vi "csmdoc_load vi description map.vi"(8 "Error In":errorcluster caption="error in (no error)", 10 "Pattern":string="VI Description(CN) - *", 11 "Path":path=path "D:/CSM Framework/Communicable-State-Machine/src/help/NEVSTOP/Communicable State Machine(CSM)") -> (0 "error out":errorcluster, 2 "NoteMap":variant, 3 "DescMap":variant)   [LabVIEW 2017, in "csmdoc.lvlib"]
doc: "### csmdoc_load vi description map.vi\n\n-- <b>Controls</b> --\n- <b>Path</b>:\n\n-- <b>Indicators</b> --\n- <b>text</b>:\n- <b>variant 2</b>:\n- <b>variant</b>:"
uses:
  csmdoc.lvlib
  Communicable State Machine.lvlib
  _Shared/CSM Shared.lvlib
panel:
  out "orders":string[](array[string])
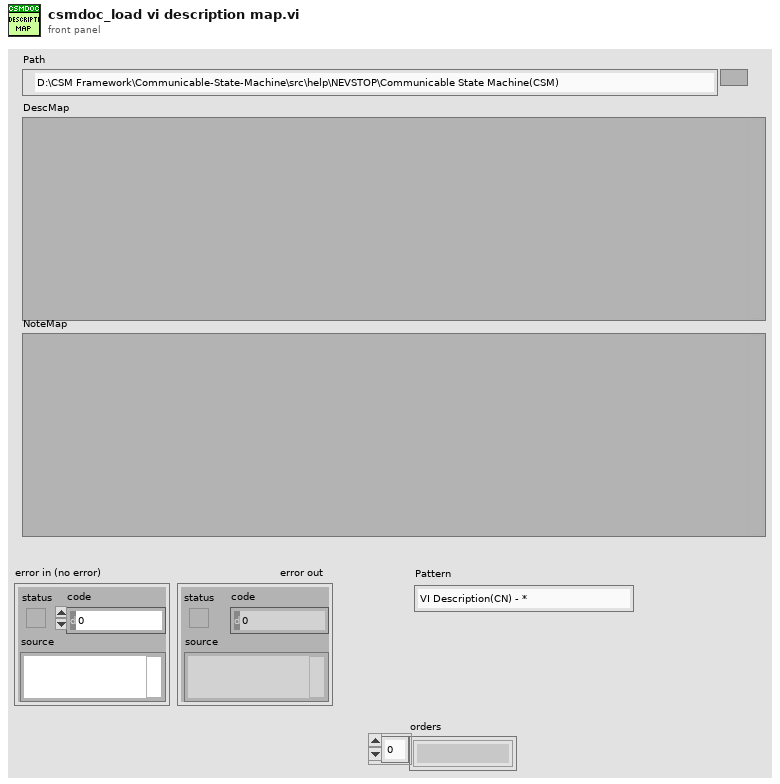
[diagram p1: front panel]
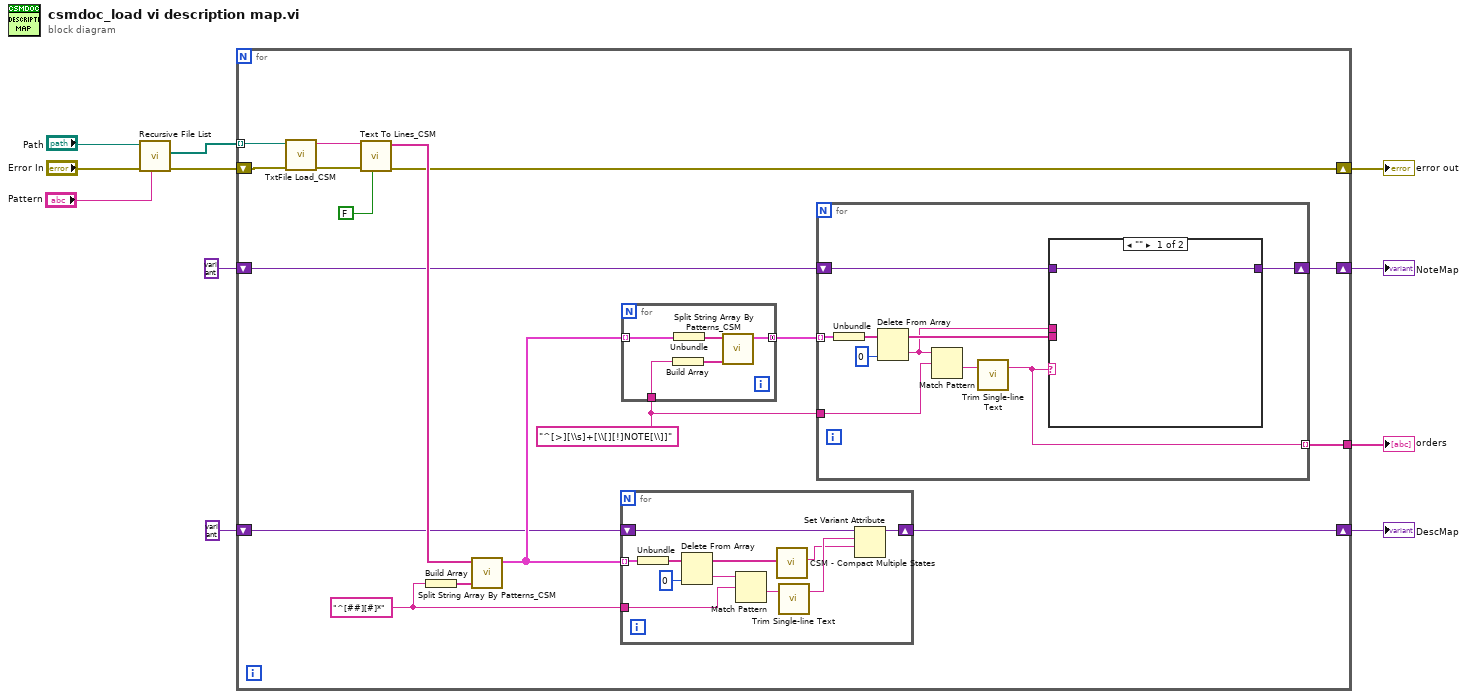
[diagram p0: block diagram]
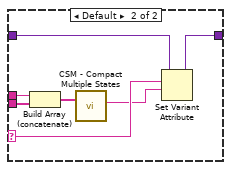
[diagram p2: hidden frame]
diagram:
  n1 = call <vilib>:"Recursive File List.vi"("pattern"="Pattern", "error in (no error)"="Error In", "Folder Path"="Path") -> ("error out"=w5:errorcluster, "All Files in Dir"=w3:path[])  [unwired: 4 in, 3 out]
  n2 = for {
    tunnel: w3 -> [w28] mode=indexing
    tunnel: [w13] -> w6
    shift-right: [w19] -> w9
    shift-left: w5 -> [w20]
    shift-right: [w14] -> w7
    shift-left: variant ("variant") -> [w17]
    shift-right: [w22] -> w11
    shift-left: variant ("variant") -> [w12]
    w15 = "^[>][\\s]+[\\[][!]NOTE[\\]]" ("delimited string")
    w24 = "^[##][#]*" ("delimited string")
    n3 = call "TxtFile Load_CSM.vi"("error in (no error)"=w20, "Path"=w28) -> ("error out"=w27:errorcluster, "Text"=w26:string)  [unwired: 8 in]
    n4 = call "Text To Lines_CSM.vi"("Remove Empty Lines? (T)"=FALSE ("Remove Empty Lines?(T)"), "error in (no error)"=w27, "String"=w26) -> ("error out"=w19:errorcluster, "Lines"=w25:string[])  [unwired: 7 in]
    n5 = Build Array(w24) -> (w23:string[])
    n6 = call "Split String Array By Patterns_CSM.vi"("Patterns"=w23, "Text Array"=w25) -> ("Array"=w18:cluster{"filtered array":string[]}[])  [unwired: 9 in]
    n7 = for {
      tunnel: w18 -> [w62] mode=indexing
      tunnel: w24 -> [w58]
      shift-right: [w52] -> w22
      shift-left: w12 -> [w53]
      n8 = Unbundle(w62) -> ("filtered array"=w61:string[])
      n9 = Delete From Array(array=w61, index=0) -> (deleted portion=w59:string, array with subset deleted=w55:string[])  [unwired: 1 in]
      n10 = Match Pattern(string=w59, regular expression=w58) -> (after substring=w57:string)  [unwired: 1 in, 3 out]
      n11 = call "CSM - Compact Multiple States.vi"("Multiple States"=w55) -> ("States"=w54:string)  [unwired: 9 in]
      n12 = call "Trim Single-line Text.vi"("single-line text"=w57) -> ("trimed text"=w56:string)  [unwired: 2 in]
      n13 = Set Variant Attribute(Variant=w53, name=w56, value=w54) -> (Variant out=w52:variant)  [unwired: 1 in, 2 out]
    }
    n14 = for {
      tunnel: w18 -> [w51] mode=indexing
      tunnel: w15 -> [w49]
      tunnel: [w47] -> w16 mode=concatenating
      n15 = Build Array(w49) -> (w48:string[])
      n16 = Unbundle(w51) -> ("filtered array"=w50:string[])
      n17 = call "Split String Array By Patterns_CSM.vi"("Patterns"=w48, "Text Array"=w50) -> ("Array"=w47:cluster{"filtered array":string[]}[])  [unwired: 9 in]
    }
    n18 = for {
      tunnel: w16 -> [w38] mode=indexing
      shift-right: [w33] -> w14
      shift-left: w17 -> [w34]
      tunnel: w15 -> [w32]
      tunnel: [w29] -> w13 mode=indexing
      n19 = Unbundle(w38) -> ("filtered array"=w37:string[])
      n20 = Delete From Array(array=w37, index=0) -> (deleted portion=w30:string, array with subset deleted=w31:string[])  [unwired: 1 in]
      n21 = Match Pattern(string=w30, regular expression=w32) -> (after substring=w35:string)  [unwired: 1 in, 3 out]
      n22 = call "Trim Single-line Text.vi"("single-line text"=w35) -> ("trimed text"=w29:string)  [unwired: 2 in]
      n23 = case shown="\"\"" w29 {
        selector: w29 -> [_ w46]
        tunnel: w34 -> [w39 w45]
        tunnel: [w39 w44] -> w33
        tunnel: w31 -> [_ w43]
        tunnel: w30 -> [_ w40]
        frame "" {
        }
        frame Default {
          n24 = Build Array (concatenate)(w40, w43) -> (w41:string[])
          n25 = call "CSM - Compact Multiple States.vi"("Multiple States"=w41) -> ("States"=w42:string)  [unwired: 9 in]
          n26 = Set Variant Attribute(Variant=w45, name=w46, value=w42) -> (Variant out=w44:variant)  [unwired: 1 in, 2 out]
        }
      }
    }
  }
  "DescMap" <- w11
  "error out" <- w9
  "NoteMap" <- w7
  "orders" <- w6
